vi "ConfigureAdaptorr01.vi"() -> ()   [LabVIEW 2011]
panel:
  out "error out":errorcluster
  out "concatenated string":string
  in  "Trip Point 1(Torr)":dbl=700.0
  in  "Set Point D (Torr)":dbl=40.0
  in  "Set Point C (Torr)":dbl=20.0
  in  "Set Point B (Torr)":dbl=76.0
  in  "Set Point A (Torr)":dbl=10.0
  in  "Trip Point 2 (Torr)":dbl=200.0
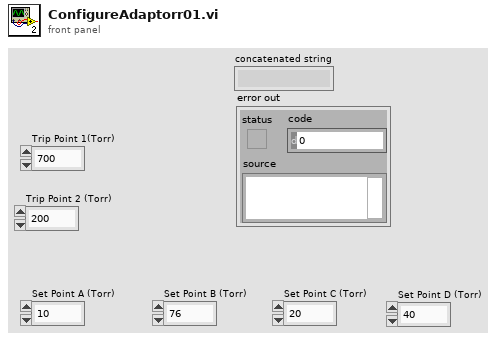
[diagram p1: front panel]
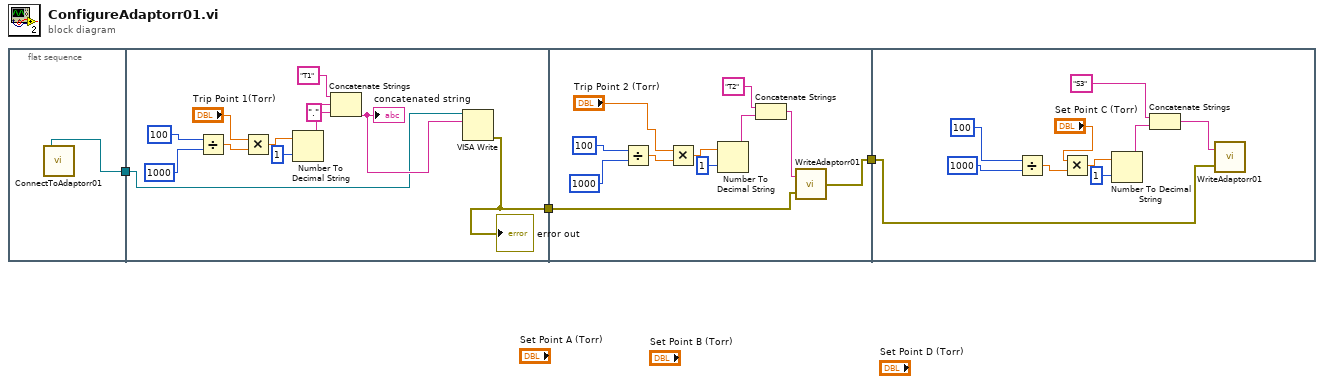
[diagram p0: block diagram]
diagram:
  n1 = flat-sequence {
    tunnel: [w4] -> w1
    tunnel: [w6] -> w2
    tunnel: w1 -> [w7]
    tunnel: [w17] -> w3
    tunnel: w2 -> [w19]
    tunnel: w3 -> [w28]
    frame #0 {
      n2 = call "ConnectToAdaptorr01.vi"() -> ("VISA resource name out"=w4:refnum<visa-resource-name>)  [unwired: 1 in, 1 out]
    }
    frame #1 {
      n3 = Divide(x=100, y=1000) -> (x/y=w14:dbl)
      n4 = Multiply(x="Trip Point 1(Torr)", y=w14) -> (x*y=w12:dbl)
      n5 = Number To Decimal String(number=w12, width (-)=i16 1) -> (decimal integer string=w9:string)
      n6 = Concatenate Strings("T1", w9, "." ("string")) -> (w8:string)
      "concatenated string" <- w8
      n7 = VISA Write(VISA resource name=w7, write buffer=w8) -> (error out=w6:errorcluster)  [unwired: 1 in, 2 out]
      "error out" <- w6
    }
    frame #2 {
      n8 = Divide(x=100, y=1000) -> (x/y=w25:dbl)
      n9 = Multiply(x="Trip Point 2 (Torr)", y=w25) -> (x*y=w24:dbl)
      n10 = Number To Decimal String(number=w24, width (-)=i16 1) -> (decimal integer string=w21:string)
      n11 = Concatenate Strings("T2", w21) -> (w18:string)
      n12 = call "WriteAdaptorr01.vi"("error in (no error)"=w19, "string to write"=w18) -> ("error out"=w17:errorcluster)
    }
    frame #3 {
      n13 = Divide(x=100, y=1000) -> (x/y=w35:dbl)
      n14 = Multiply(x="Set Point C (Torr)", y=w35) -> (x*y=w32:dbl)
      n15 = Number To Decimal String(number=w32, width (-)=i16 1) -> (decimal integer string=w30:string)
      n16 = Concatenate Strings("S3", w30) -> (w29:string)
      n17 = call "WriteAdaptorr01.vi"("error in (no error)"=w28, "string to write"=w29) -> ()  [unwired: 1 out]
    }
  }
